vi "Get Input Kinds.vi"(8 "error in (no error)":errorcluster, 11 "OBS in":refnum<class "OBS.lvclass">) -> (0 "error out":errorcluster, 2 "Input Kinds":string[](array[string]), 3 "OBS out":refnum<class "OBS.lvclass">)   [LabVIEW 2020, in "obs-websocket.lvlib" / "OBS.lvclass"]
uses:
  OBS.lvclass
  GetInputKindList/GetInputKindList.lvclass
  C:/dev/lv20CE/relink/lv-obs-websocket/obs-websocket/Client Message/Client Message.lvclass
  RGetInputKindList/RGetInputKindList.lvclass
  C:/dev/lv20CE/relink/lv-obs-websocket/obs-websocket/Response/Response.lvclass
  OBS.lvclass/OBS.ctl
  C:/dev/lv20CE/relink/lv-obs-websocket/obs-websocket/Server Message/Server Message.lvclass
  C:/dev/lv20CE/relink/lv-obs-websocket/obs-websocket/Message/Message.lvclass
  C:/dev/lv20CE/relink/lv-promises/Promises/Value/Value.lvclass
  C:/dev/lv20CE/relink/lv-obs-websocket/obs-websocket/RGetInputKindList/RGetInputKindList.lvclass
  C:/dev/lv20CE/relink/lv-obs-websocket/obs-websocket/Request/Request.lvclass
  C:/dev/lv20CE/relink/lv-obs-websocket/obs-websocket/GetInputKindList/GetInputKindList.lvclass
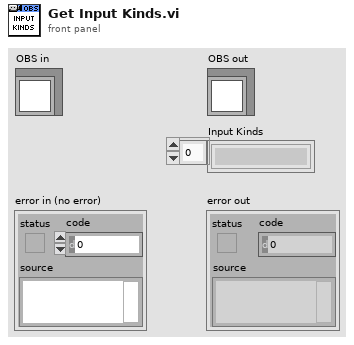
[diagram p1: front panel]
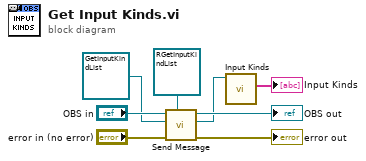
[diagram p0: block diagram]
diagram:
  n1 = call "Send Message.vi"("Response Type (None)"=refnum<class "RGetInputKindList.lvclass"> refnum ("obs-websocket.lvlib:RGetInputKindList.lvclass"), "error in (no error)"="error in (no error)", "Client Message"=refnum<class "GetInputKindList.lvclass"> refnum ("obs-websocket.lvlib:GetInputKindList.lvclass"), "OBS in"="OBS in") -> ("error out"=→"error out":errorcluster, "Response"=w2:refnum<class "RGetInputKindList.lvclass">, "OBS out"=→"OBS out":refnum<class "OBS.lvclass">)  [unwired: 4 in, 1 out]
  n2 = call "Input Kinds.vi"("RGetInputKindList in"=w2) -> ("Input Kinds"=→"Input Kinds":string[])  [unwired: 8 in, 2 out]
